vi "Reset.vi"(8 "error in (no error)":errorcluster, 11 "SLSC Switch in":refnum<class "SLSC Switch.lvclass">) -> (0 "error out":errorcluster, 3 "SLSC Switch out":refnum<class "SLSC Switch.lvclass">)   [LabVIEW 2015, in "SLSC Switch.lvlib" / "SLSC Switch.lvclass"]
doc: "Opens all relays."
uses:
  SLSC Switch.lvclass
  slscsl/RelayAction.ctl
  Controls/Connection.ctl
  SLSC Switch.lvclass/SLSC Switch.ctl
  Switch Action Processor/Switch Action Processor.lvclass/Switch Action Processor.ctl
  Relay/Relay.lvclass/Relay.ctl
  Relay/Read name.vi
  Switch Action Processor/Read Relays.vi
  <vilib>/SLSC/Flatten Names (String).vi
  Relay/Relay.lvclass
  slscsl/slscsl.lvclass
  <vilib>/SLSC/SLSC.lvlib
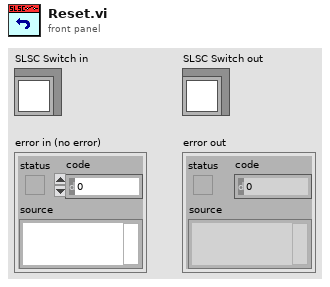
[diagram p1: front panel]
types:
  T1 = typedef "SLSC Switch.lvlib/SLSC Switch.lvclass/Connection.ctl" = cluster{"channel 1":string, "channel 2":string}
  T2 = typedef "SLSC Switch.lvlib/slscsl.lvclass/RelayAction.ctl" = u32
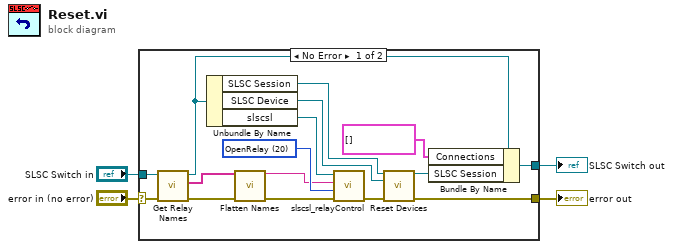
[diagram p0: block diagram]
diagram:
  n1 = case shown="No Error" "error in (no error)" {
    selector: "error in (no error)" -> [w12 w22]
    tunnel: [w6 w22] -> w3
    tunnel: [w15 w21] -> w1
    tunnel: "SLSC Switch in" -> [w20 w21]
    frame No Error {
      w18 = T2 20 items=["CloseRelay"=21, "OpenRelay"=20] ("RelayAction")
      n2 = call "Get Relay Names.vi"("error in (no error)"=w12, "SLSC Switch in"=w20) -> ("error out"=w11:errorcluster, "Relay Names"=w14:string[], "SLSC Switch out"=w17:refnum<class "SLSC Switch.lvclass">)  [unwired: 7 in]
      n3 = Unbundle By Name(w17) -> ("SLSC Session"=w9:refnum<k21>, "SLSC Device"=w8:refnum<k21>, "slscsl"=w19:refnum<class "slscsl.lvclass">)
      n4 = call-poly <vilib>:"Flatten Names.vi"("names in"=w14, "error in (no error)"=w11) -> ("names out"=w13:string, "error out"=w10:errorcluster)  [unwired: 12 in]
      n5 = call "slscsl_relayControl.vi"("error in (no error)"=w10, "RelayAction"=w18, "relayNames"=w13, "slscsl in"=w19) -> ("error out"=w7:errorcluster)  [unwired: 5 in, 2 out]
      n6 = call <vilib>:"Reset Devices.vi"("session in"=w9, "devices"=w8, "error in (no error)"=w7) -> ("session out"=w5:refnum<k21>, "error out"=w6:errorcluster)  [unwired: 11 in]
      n7 = Bundle By Name(cluster=w17, "Connections"=T1[] [], "SLSC Session"=w5) -> (w15:refnum<class "SLSC Switch.lvclass">)
    }
    frame Error {
    }
  }
  "error out" <- w3
  "SLSC Switch out" <- w1
